vi "Load Config.vi"(6 "Constants":refnum<class "Sequence Constants.lvclass">, 8 "error in (no error)":refnum<class "MultiErrors.lvclass">, 10 "Config Element":refnum<class "Config Element.lvclass">, 11 "Reset Var Command Config in":refnum<class "Reset Var Command Config.lvclass">) -> (0 "error out":refnum<class "MultiErrors.lvclass">, 3 "Reset Var Command Config out":refnum<class "Reset Var Command Config.lvclass">)   [LabVIEW 2020, in "VolatusSeqConfig.lvlib" / "Reset Var Command Config.lvclass"]
uses:
  Reset Var Command Config.lvclass
  VolatusErrorUtilities/MultiErrors/MultiErrors.lvclass
  lv-cdm/CDM-Config/Config Element/Config Element.lvclass
  Sequence Constants/Sequence Constants.lvclass
  Reset Var Command Config.lvclass/Reset Var Command Config.ctl
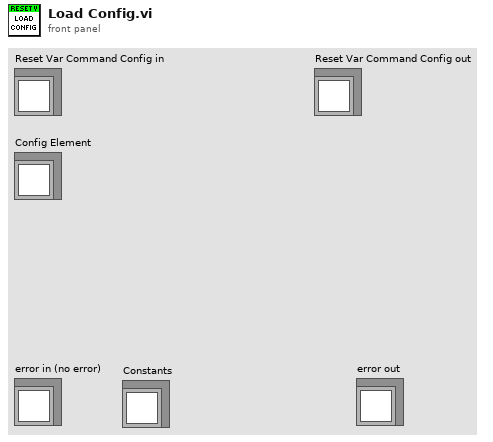
[diagram p1: front panel]
types:
  T1 = typedef "CDM-Config.lvlib/Value Type.ctl" = enum16{"String", "Number", "Bool", "Object", "Array"}
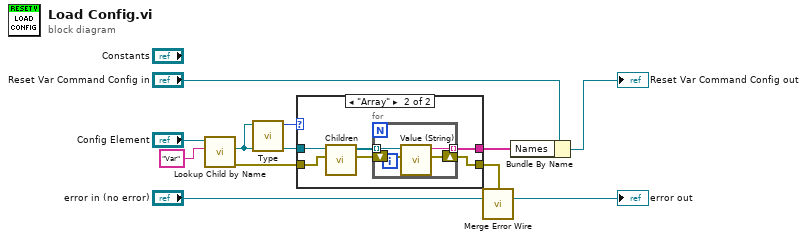
[diagram p0: block diagram]
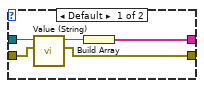
[diagram p2: hidden frame]
diagram:
  n1 = call "Lookup Child by Name.vi"("Name"="Var", "Config Element in"="Config Element") -> ("error out"=w6:errorcluster, "Child"=w7:refnum<class "Config Element.lvclass">)  [unwired: 6 in, 2 out]
  n2 = call "Type.vi"("Config Element in"=w7) -> ("Value Type"=w8:T1)  [unwired: 9 in, 1 out]
  n3 = case shown="\"Array\"" w8 {
    tunnel: w7 -> [w16 w22]
    tunnel: w6 -> [w15 w21]
    tunnel: [w13 w18] -> w1
    tunnel: [w12 w17] -> w4
    frame Default {
      n4 = call "Value (String).vi"("error in (no error)"=w15, "Config Element in"=w16) -> ("error out"=w12:errorcluster, "String Value"=w14:string)  [unwired: 8 in]
      n5 = Build Array(w14) -> (w13:string[])
    }
    frame "Array" {
      n6 = call "Children.vi"("error in (no error)"=w21, "Config Element in"=w22) -> ("error out"=w20:errorcluster, "Elements"=w19:refnum<class "Config Element.lvclass">[])  [unwired: 8 in]
      n7 = for {
        shift-right: [w24] -> w17
        shift-left: w20 -> [w25]
        tunnel: w19 -> [w26] mode=indexing
        tunnel: [w23] -> w18 mode=indexing
        n8 = call "Value (String).vi"("error in (no error)"=w25, "Config Element in"=w26) -> ("error out"=w24:errorcluster, "String Value"=w23:string)  [unwired: 8 in]
      }
    }
  }
  n9 = call "Merge Error Wire.vi"("error in (no error)"=w4, "MultiErrors in"="error in (no error)") -> ("MultiErrors out"=→"error out":refnum<class "MultiErrors.lvclass">)  [unwired: 13 in]
  n10 = Bundle By Name(cluster="Reset Var Command Config in", "Names"=w1) -> (→"Reset Var Command Config out":refnum<class "Reset Var Command Config.lvclass">)
